vi "add_data_line#_exp.vi"(8 "error in (no error)":errorcluster, 9 "#":i32=-1, 10 "add Array":sgl[](array[numeric]), 11 "Experiment.lvclass in":refnum<class "Experiment.lvclass">) -> (0 "error out":errorcluster, 3 "Experiment.lvclass out":refnum<class "Experiment.lvclass">)   [LabVIEW 2018, in "Experiment.lvclass"]
uses:
  Experiment.lvclass
  Experiment.lvclass/Experiment.ctl
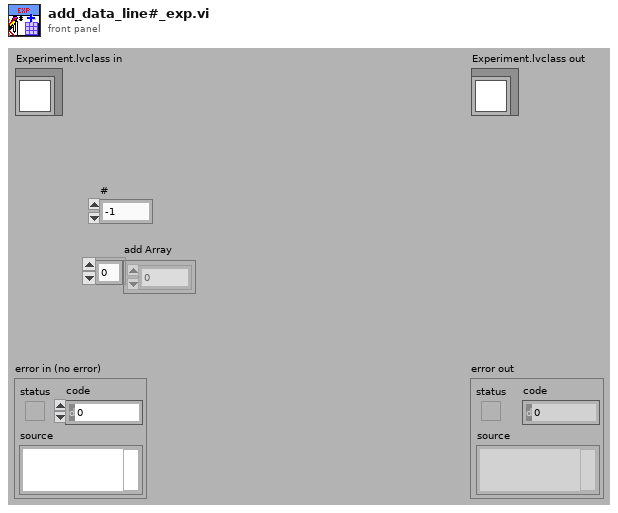
[diagram p1: front panel]
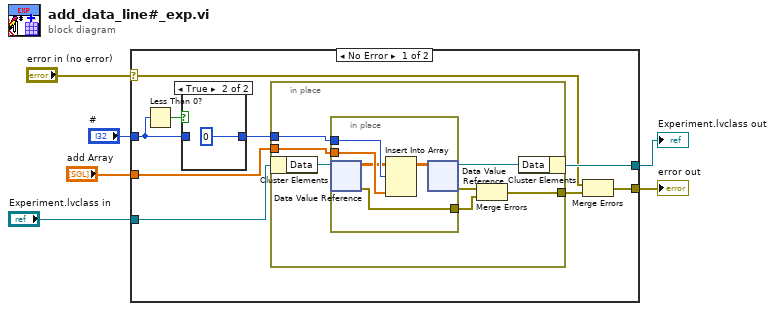
[diagram p0: block diagram]
diagram:
  n1 = case shown="No Error" "error in (no error)" {
    selector: "error in (no error)" -> [w9 w30]
    tunnel: [w8 w30] -> w5
    tunnel: [w13 w31] -> w3
    tunnel: "Experiment.lvclass in" -> [w14 w31]
    tunnel: "add Array" -> [w15 _]
    tunnel: "#" -> [w12 _]
    frame No Error {
      n2 = Less Than 0?(x=w12) -> (x < 0?=w11:bool)
      n3 = case shown="True" w11 {
        tunnel: w12 -> [w16 _]
        tunnel: [w16 0] -> w10
        frame False {
        }
        frame True {
        }
      }
      n4 = in-place {
        in-place-border: w15 -> [w22]
        in-place-border: w10 -> [w23]
        in-place-border: [w18] -> w7
        n5 = in-place-cluster #1(w14) -> ("Data"=w24:refnum<data-value>)
        n6 = in-place {
          in-place-border: w23 -> [w29]
          in-place-border: w22 -> [w28]
          in-place-border: [w25] -> w20
          n7 = in-place-dvr #2(w24) -> (w27:sgl[][], w25:errorcluster)
          n8 = Insert Into Array(array=w27, index (row)=w29, new element=w28) -> (w26:sgl[][])  [unwired: 1 in]
          n9 = in-place-dvr #2(w26) -> (w21:refnum<data-value>, w19:errorcluster)
        }
        n10 = Merge Errors(w19, w20) -> (w18:errorcluster)
        n11 = in-place-cluster #1("Data"=w21) -> (w13:refnum<class "Experiment.lvclass">)
      }
      n12 = Merge Errors(w9, w7) -> (w8:errorcluster)
    }
    frame Error {
    }
  }
  "error out" <- w5
  "Experiment.lvclass out" <- w3
